vi "run.vi"(8 "error in (no error)":errorcluster, 11 "DataCollectionDL110128Streaming in":refnum<class "DataCollectionDL110128Streaming.lvclass">) -> (0 "error out":errorcluster, 3 "DataCollectionDL110128Streaming out":refnum<class "DataCollectionDL110128Streaming.lvclass">)   [LabVIEW 2010, in "DataCollectionDL110128Streaming.lvclass"]
uses:
  DataCollectionDL110128Streaming.lvclass
  common/xcontrols/XSettings/XSettings/XSettings.xctl
  common/classes/GenericComponent/GenericComponent/GenericComponent.lvclass
  DataCollectionDL110128Streaming.lvclass/DataCollectionDL110128Streaming.ctl
  DataCollectionDL091104Scaffold/DataCollectionDL091104Scaffold/DataCollectionDL091104Scaffold.lvclass
  common/classes/ErrorController/ErrorController/class_data.vi
  common/classes/ErrorController/ErrorController/ErrorController.lvclass
  GenericDataCollection/GenericDataCollection/GenericDataCollection.lvclass
panel:
  in  "Tab Control":enum32{"User", "Debug", "About"}(tab)
  in  "autosave?":bool
  in  "XSettings":refnum<class "GenericComponent.lvclass">(xcontrol)
  out "loaded settings?":bool
  out "finished?":bool
  # "DataCollectionDL110128Streaming\n\nAuthors: Andreas Keller and Dominik Langer, ETH Zurich, Switzerland"
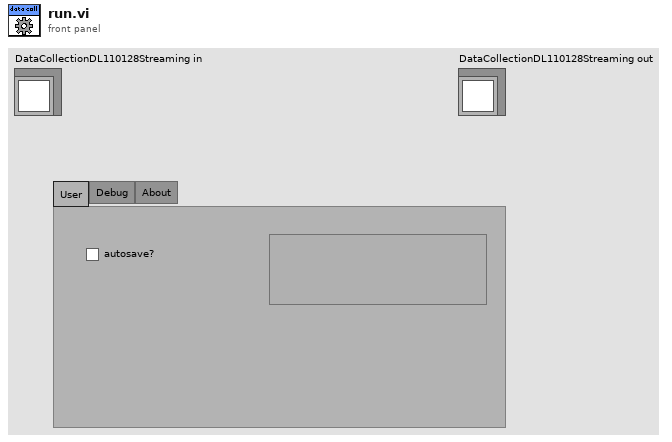
[diagram p1: front panel]
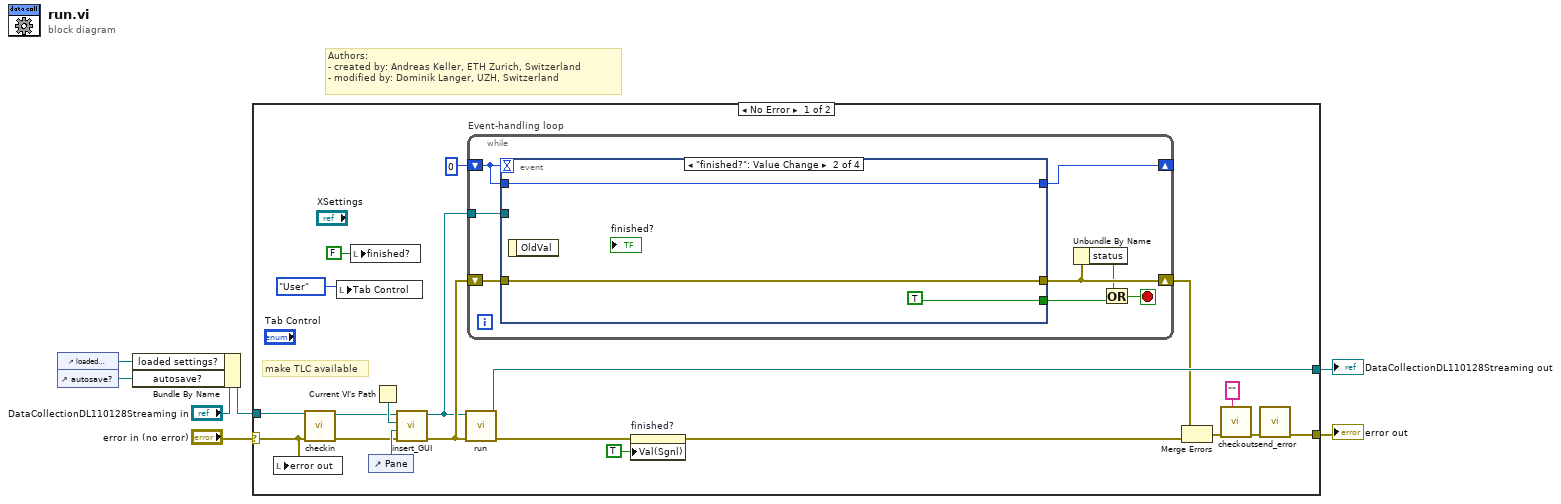
[diagram p0: block diagram]
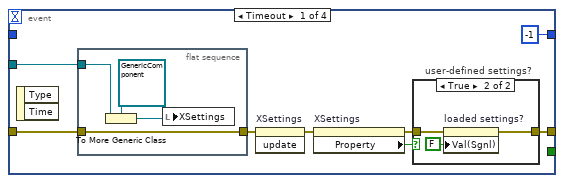
[diagram p2: hidden frame]
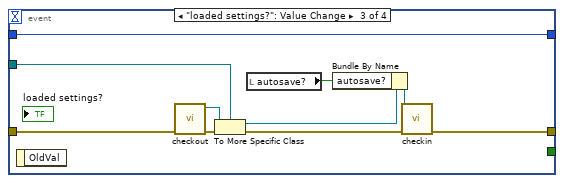
[diagram p4: hidden frame]
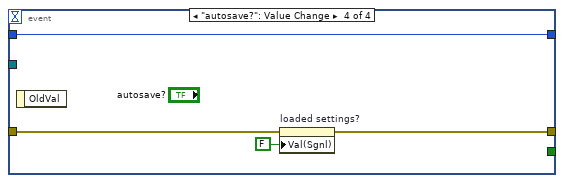
[diagram p5: hidden frame]
diagram:
  # "Authors: \n- created by: Andreas Keller, ETH Zurich, Switzerland\n- modified by: Dominik Langer, UZH, Switzerland"
  n1 = control-ref of="loaded settings?"() -> (w1:refnum<vi>)
  n2 = control-ref of="autosave?"() -> (w2:refnum<vi>)
  n3 = Bundle By Name(cluster="DataCollectionDL110128Streaming in", "loaded settings?"=w1, "autosave?"=w2) -> (w3:refnum<class "DataCollectionDL110128Streaming.lvclass">)
  n4 = case shown="No Error" "error in (no error)" {
    selector: "error in (no error)" -> [w21 w70]
    tunnel: [w27 w70] -> w7
    tunnel: w3 -> [w23 w69]
    tunnel: [w20 w69] -> w6
    frame No Error {
      # "make TLC available"
      n5 = local write "error out"(w21) -> ()
      n6 = call-dynamic "checkin.vi"("error in (no error)"=w21, "GenericDataCollection in"=w23) -> ("error out"=w18:errorcluster, "GenericDataCollection out"=w19:refnum<class "DataCollectionDL110128Streaming.lvclass">)  [unwired: 8 in]
      n7 = local write "Tab Control"(enum32{"User", "Debug", "About"}."User" ("Tab Control")) -> ()
      n8 = local write "finished?"(FALSE ("finished?")) -> ()
      n9 = control-ref of="Pane"() -> (w24:refnum<vi>)
      n10 = Current VI's Path() -> (path=w25:path)
      n11 = call-dynamic "insert_GUI.vi"("error in (no error)"=w18, "Pane"=w24, "VI path"=w25, "GenericComponent in"=w19) -> ("error out"=w17:errorcluster, "GenericComponent out"=w16:refnum<class "DataCollectionDL110128Streaming.lvclass">)  [unwired: 6 in]
      n12 = call-parent "run.vi"("error in (no error)"=w17, "DataCollectionDL091104Scaffold.lvclass out"=w16) -> ("error out"=w9:errorcluster, "DataCollectionDL091104Scaffold.lvclass out"=w20:refnum<class "DataCollectionDL110128Streaming.lvclass">)  [unwired: 8 in]
      n13 = while "Event-handling loop" {
        shift-right: [w34] -> w14
        shift-left: w17 -> [w35]
        tunnel: w16 -> [w30]
        shift-right: [w28] -> _
        shift-left: 0 -> [w29]
        stop <- w33 stop-if-true
        n14 = event shown="[1] \"finished?\": Value Change" {
          selector: _ -> [_ _ _ _]
          dyn-events: _ -> [_ _ _ _]
          timeout: w29 -> [_ _ _ _]
          tunnel: w35 -> [w42 w54 w64 w68]
          tunnel: [w38 w54 w63 w67] -> w34
          tunnel: [_ TRUE _ _] -> w32
          tunnel: w30 -> [w43 _ w62 _]
          tunnel: w29 -> [_ w52 w55 w65]
          tunnel: [-1 w52 w55 w65] -> w28
          event Timeout {
            n15 = event-data() -> ()  [unwired: 1 in, 2 out]
            n16 = flat-sequence {
              tunnel: w43 -> [w51]
              tunnel: w42 -> [w48]
              tunnel: [w48] -> w41
              frame #0 {
                n17 = To More Generic Class(target class=refnum<class "GenericComponent.lvclass"> refnum ("GenericComponent.lvclass"), reference=w51) -> (generic class reference=w49:refnum<class "GenericComponent.lvclass">)
                n18 = local write "XSettings"(w49) -> ()
              }
            }
            n19 = invoke on="XSettings" class="XSettings (strict)" method="update"(error in=w41) -> (error out=w40:errorcluster)  [unwired: 2 in, 2 out]
            n20 = property on="XSettings" class="XSettings (strict)"(error in=w40) -> (error out=w39:errorcluster, "Property"=w37:bool)  [unwired: 1 in, 1 out]
            n21 = case "user-defined settings?" shown="True" w37 {
              tunnel: w39 -> [w44 w47]
              tunnel: [w44 w46] -> w38
              frame False {
              }
              frame True {
                n22 = property on="loaded settings?" class="Bool (strict)"(error in=w47, "Val(Sgnl)"=FALSE ("Value (Signaling)")) -> (error out=w46:errorcluster)  [unwired: 1 in, 1 out]
              }
            }
          }
          event "finished?": Value Change {
            n23 = event-data() -> ()  [unwired: 1 in, 1 out]
          }
          event "loaded settings?": Value Change {
            n24 = event-data() -> ()  [unwired: 1 in, 1 out]
            n25 = call "checkout.vi"("error in (no error)"=w64) -> ("error out"=w60:errorcluster, "GenericDataCollection out"=w61:refnum<class "GenericDataCollection.lvclass">)  [unwired: 9 in]
            n26 = To More Specific Class(target class=w62, reference=w61, error in=w60) -> (specific class reference=w58:refnum<class "DataCollectionDL110128Streaming.lvclass">, error out=w59:errorcluster)
            n27 = local read "autosave?"() -> (w56:bool)
            n28 = Bundle By Name(cluster=w58, "autosave?"=w56) -> (w57:refnum<class "DataCollectionDL110128Streaming.lvclass">)
            n29 = call-dynamic "checkin.vi"("error in (no error)"=w59, "GenericDataCollection in"=w57) -> ("error out"=w63:errorcluster)  [unwired: 8 in, 1 out]
          }
          event "autosave?": Value Change {
            n30 = event-data() -> ()  [unwired: 1 in, 1 out]
            n31 = property on="loaded settings?" class="Bool (strict)"(error in=w68, "Val(Sgnl)"=FALSE ("Value (Signaling)")) -> (error out=w67:errorcluster)  [unwired: 1 in, 1 out]
          }
        }
        n32 = Unbundle By Name(w34) -> ("status"=w31:bool)
        n33 = Or(x=w31, y=w32) -> (x .or. y?=w33:bool)
      }
      n34 = property on="finished?" class="Bool (strict)"(error in=w9, "Val(Sgnl)"=TRUE ("Value (Signaling)")) -> (error out=w8:errorcluster)  [unwired: 1 in, 1 out]
      n35 = Merge Errors(w14, w8) -> (w13:errorcluster)
      n36 = call "checkout.vi"("locked by?"="", "error in (no error)"=w13) -> ("error out"=w12:errorcluster)  [unwired: 8 in, 1 out]
      n37 = call "send_error.vi"("error in (no error)"=w12) -> ("error out"=w27:errorcluster)  [unwired: 10 in]
    }
    frame Error {
    }
  }
  "error out" <- w7
  "DataCollectionDL110128Streaming out" <- w6
